vi "receive.vi"(8 "error in (no error)":errorcluster, 11 "Test Redis Client in":refnum<class "Test Redis Client.lvclass">) -> (0 "error out":errorcluster, 1 "timed out?":bool, 2 "RESP3 Value":variant, 3 "Test Redis Client out":refnum<class "Test Redis Client.lvclass">)   [LabVIEW 2019, in "Test Redis Client for LabVIEW.lvlib" / "Test Redis Client.lvclass"]
uses:
  Test Redis Client.lvclass
  lib/RESP3-for-LabVIEW/RESP3/RESP3 Parser/RESP3 Parser.lvclass
  Test Redis Client.lvclass/Test Redis Client.ctl
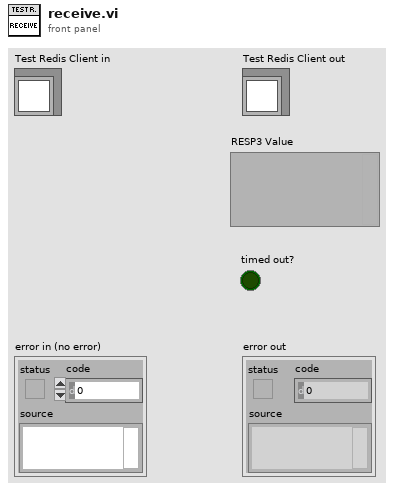
[diagram p1: front panel]
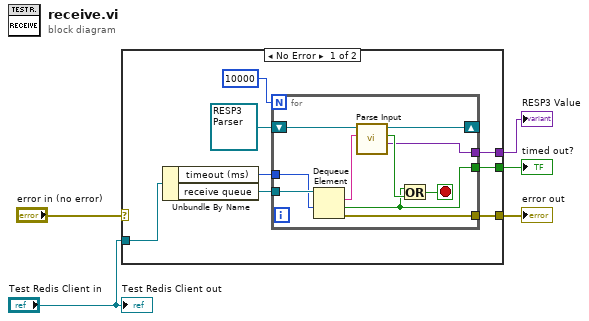
[diagram p0: block diagram]
diagram:
  n1 = case shown="No Error" "error in (no error)" {
    selector: "error in (no error)" -> [_ w24]
    tunnel: "Test Redis Client in" -> [w13 _]
    tunnel: [w11 w24] -> w4
    tunnel: [w10 _] -> w2
    tunnel: [w6 _] -> w1
    frame No Error {
      n2 = Unbundle By Name(w13) -> ("timeout (ms)"=w9:i32, "receive queue"=w12:refnum<queue>)
      n3 = for {
        N: 10000 -> [_]
        tunnel: w12 -> [w23]
        tunnel: [w22] -> w11
        tunnel: [w14] -> w10
        tunnel: w9 -> [w21]
        shift-right: [w19] -> _
        shift-left: refnum<class "RESP3 Parser.lvclass"> refnum ("RESP3.lvlib:RESP3 Parser.lvclass") -> [w20]
        tunnel: [w16] -> w6
        stop <- w15 stop-if-true
        n4 = Dequeue Element(queue=w23, timeout in ms (-1)=w21) -> (element=w17:string, timed out?=w14:bool, error out=w22:errorcluster)  [unwired: 1 in, 1 out]
        n5 = call-dynamic "Parse Input.vi"("input line"=w17, "RESP3 Parser in"=w20) -> ("RESP3 Value"=w16:variant, "finished?"=w18:bool, "RESP3 Parser out"=w19:refnum<class "RESP3 Parser.lvclass">)  [unwired: 5 in, 2 out]
        n6 = Or(x=w14, y=w18) -> (x .or. y?=w15:bool)
      }
    }
    frame Error {
    }
  }
  "error out" <- w4
  "timed out?" <- w2
  "RESP3 Value" <- w1
  "Test Redis Client out" <- "Test Redis Client in"
